vi "Capacitor to Sweep to Register to Write.vi"(8 "error in (no error)":errorcluster, 11 "Toggle 7.1 in":refnum<class "Toggle 7.1.lvclass">) -> (0 "error out":errorcluster, 1 "Cap Value Array":cluster{"Register Number":u32, "Value":dbl}[](array[cluster]), 2 "Cap Register Array":T1[](array[typedef]), 3 "Toggle 7.1 out":refnum<class "Toggle 7.1.lvclass">)   [LabVIEW 2020, in "Toggle 7.1.lvclass"]
uses:
  Toggle 7.1.lvclass
  Controls/Register to Write.ctl
  PIC-device/PIC-Device.lvclass
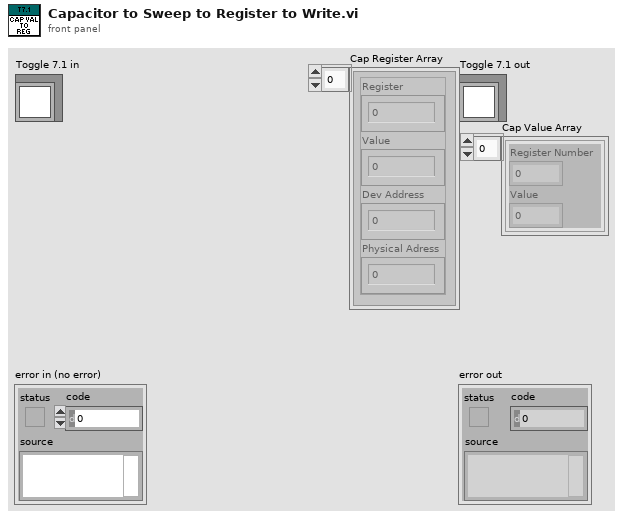
[diagram p1: front panel]
types:
  T1 = typedef "PIC-Device.lvclass/Register to Write.ctl" = cluster{"Register":u32, "Value":u32, "Dev Address":u32, "Physical Adress":u32}
  T2 = typedef "Toggle 7.1.lvclass/Parameter Cluster.ctl" = cluster{"Enable":bool, "Register Number":u32, "Use Array":bool, "Array":dbl[], "To From Cluster":cluster{"From":dbl, "To":dbl, "Step":dbl}}
  T3 = typedef "Toggle 7.1.lvclass/Capacitor register.ctl" = cluster{"Register":u32, "Beam":dbl, "Trimmers":dbl[]}
  T4 = cluster{"Register Number":u32, "Numeric Control":dbl}
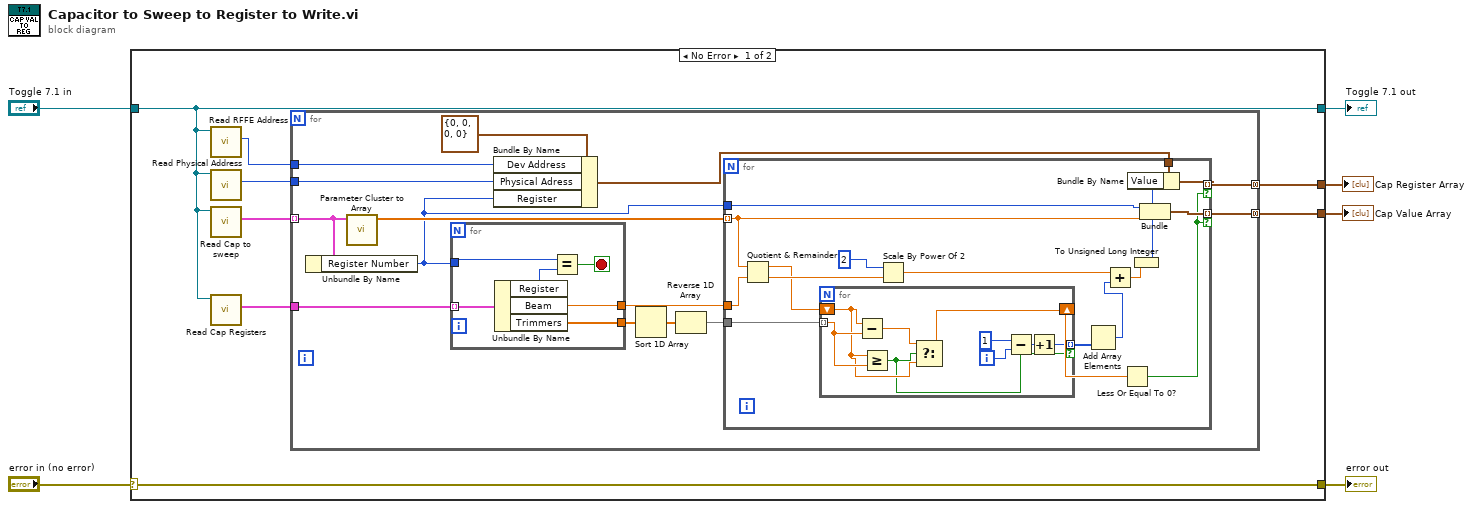
[diagram p0: block diagram]
diagram:
  n1 = case shown="No Error" "error in (no error)" {
    selector: "error in (no error)" -> [w14 w62]
    tunnel: [w14 w62] -> w5
    tunnel: [w11 w61] -> w3
    tunnel: "Toggle 7.1 in" -> [w11 w61]
    tunnel: [w8 _] -> w2
    tunnel: [w7 _] -> w1
    frame No Error {
      n2 = call-dynamic "Read RFFE Address.vi"("Toggle 6 in"=w11) -> ("RFFE Adress"=w10:u32)  [unwired: 8 in, 2 out]
      n3 = call-dynamic "Read Physical Address.vi"("Toggle 6 in"=w11) -> ("Physical Adress"=w9:u32)  [unwired: 9 in, 1 out]
      n4 = call-dynamic "Read Cap to sweep.vi"("Toggle 6 in"=w11) -> ("Cap to sweep"=w13:T2[])  [unwired: 9 in, 1 out]
      n5 = call-dynamic "Read Cap Registers.vi"("Toggle 6 in"=w11) -> ("Cap Registers"=w12:T3[])  [unwired: 9 in, 1 out]
      n6 = for {
        tunnel: w13 -> [w28] mode=indexing
        tunnel: w12 -> [w27]
        tunnel: w10 -> [w22]
        tunnel: w9 -> [w21]
        tunnel: [w18] -> w8 mode=concatenating
        tunnel: [w17] -> w7 mode=concatenating
        n7 = Unbundle By Name(w28) -> ("Register Number"=w19:u32)
        n8 = call "Parameter Cluster to Array.vi"("Parameter Cluster"=w28) -> ("Array"=w26:dbl[])  [unwired: 10 in]
        n9 = for {
          tunnel: w19 -> [w58]
          tunnel: w27 -> [w60] mode=indexing
          tunnel: [w56] -> w25
          tunnel: [w55] -> w24
          stop <- w57 stop-if-true
          n10 = Unbundle By Name(w60) -> ("Register"=w59:u32, "Beam"=w56:dbl, "Trimmers"=w55:dbl[])
          n11 = Equal?(x=w58, y=w59) -> (x = y?=w57:bool)
        }
        n12 = Bundle By Name(cluster=T1 {"Register"=0, "Value"=0, "Dev Address"=0, "Physical Adress"=0} ("Register to Write"), "Dev Address"=w22, "Physical Adress"=w21, "Register"=w19) -> (w20:T1)
        n13 = Sort 1D Array(array=w24) -> (sorted array=w16:dbl[])
        n14 = Reverse 1D Array(array=w16) -> (reversed array=w15:dbl[])
        n15 = for {
          tunnel: w26 -> [w40] mode=indexing
          tunnel: w25 -> [w45]
          tunnel: w15 -> [w33]
          tunnel: w20 -> [w38]
          tunnel: w19 -> [w41]
          tunnel: [w39] -> w17 mode=indexing if=w29
          tunnel: [w35] -> w18 mode=indexing if=w29
          n16 = Quotient & Remainder(x=w40, y=w45) -> (x-y*floor(x/y)=w34:dbl, floor(x/y)=w43:dbl)
          n17 = for {
            shift-right: [w51] -> w30
            shift-left: w34 -> [w52]
            tunnel: w33 -> [w53] mode=indexing
            tunnel: [w46] -> w32 mode=indexing if=w47
            i -> [w49]
            n18 = Subtract(x=w52, y=w53) -> (x-y=w54:dbl)
            n19 = Greater Or Equal?(x=w52, y=w53) -> (x >= y?=w47:bool)
            n20 = Select(t=w54, s=w47, f=w52) -> (s? t:f=w51:dbl)
            n21 = Subtract(x=1, y=w49) -> (x-y=w48:i32)
            n22 = Increment(x=w48) -> (x+1=w46:i32)
          }
          n23 = Scale By Power Of 2(n=i16 2, x=w43) -> (x*2^n=w42:dbl)
          n24 = Add Array Elements(numeric array=w32) -> (sum=w31:i32)
          n25 = Add(x=w42, y=w31) -> (x+y=w37:dbl)
          n26 = Less Or Equal To 0?(x=w30) -> (x <= 0?=w29:bool)
          n27 = To Unsigned Long Integer(number=w37) -> (unsigned 32bit integer=w36:u32)
          n28 = Bundle By Name(cluster=w38, "Value"=w36) -> (w35:T1)
          n29 = Bundle("Register Number"=w41, "Numeric Control"=w40) -> (w39:T4)  [unwired: 1 in]
        }
      }
    }
    frame Error {
    }
  }
  "error out" <- w5
  "Toggle 7.1 out" <- w3
  "Cap Register Array" <- w2
  "Cap Value Array" <- w1
